vi "Lexer.vi"(8 "error in (no error)":errorcluster, 11 "Input":string) -> (0 "error out":errorcluster, 3 "Tokens":T1[](array[typedef]))   [LabVIEW 2022 SP3, in "Expressions.lvlib"]
uses:
  Expressions.lvlib
  Controls/Token.ctl
  Controls/Token Type.ctl
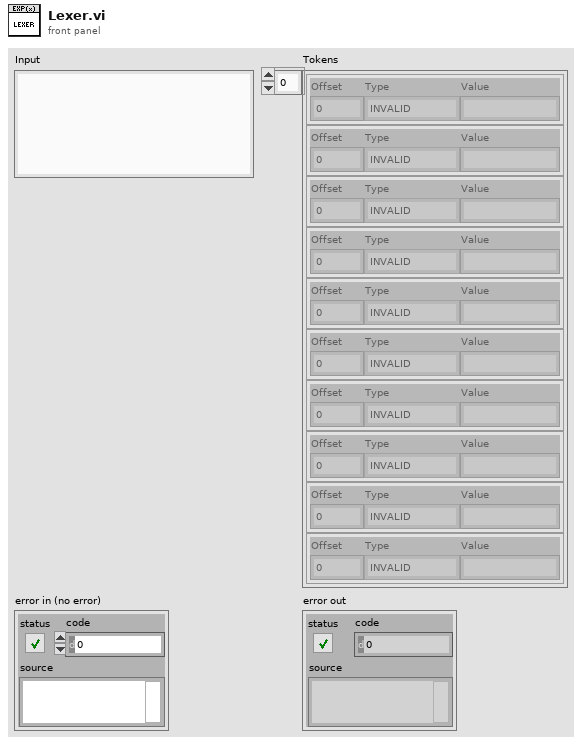
[diagram p1: front panel]
types:
  T1 = typedef "Expressions.lvlib/Token.ctl" = cluster{"Offset":i32, "Type":T2, "Value":string}
  T2 = typedef "Expressions.lvlib/Token Type.ctl" = enum8{"INVALID", "NOT", "AND", "OR", "EE", "NE", "LT", "GT", "LTE", "GTE", "PLUS", "MINUS", "MULTIPLY", "DIVIDE", "MODULUS", "LPAREN", "RPAREN", "LITERAL", "IDENTIFIER", "DEFINITION"}
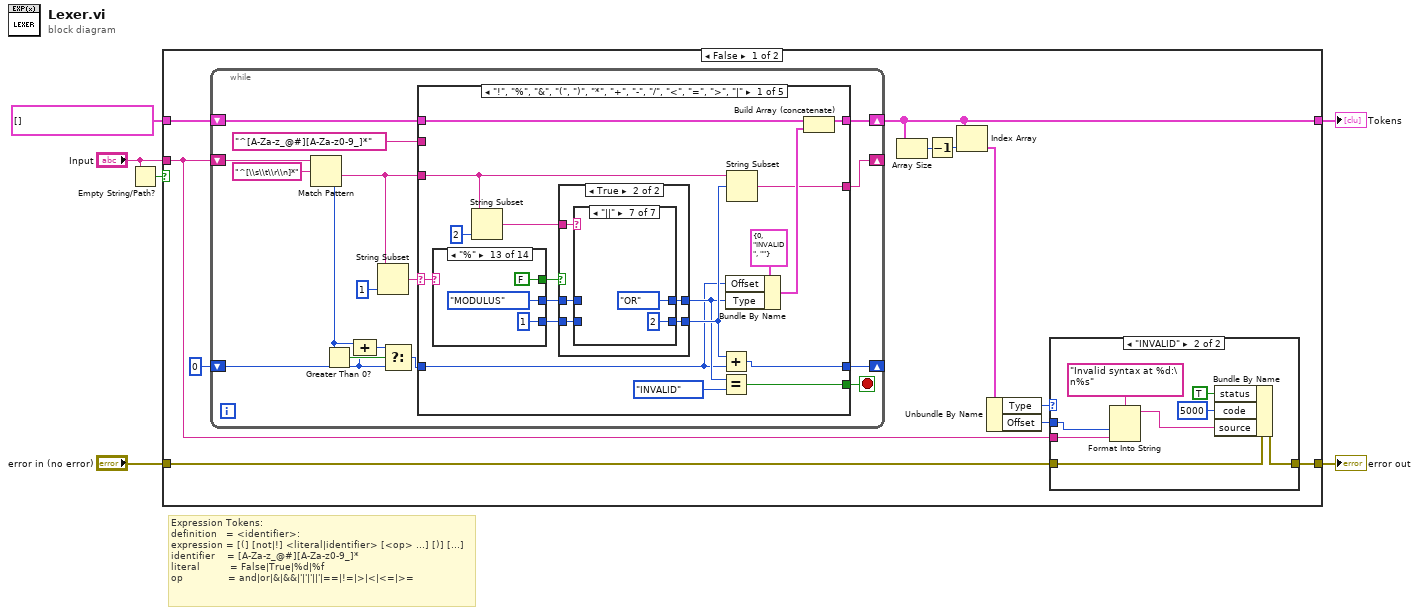
[diagram p0: block diagram]
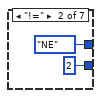
[diagram p5: hidden frame]
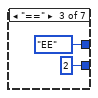
[diagram p6: hidden frame]
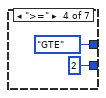
[diagram p7: hidden frame]
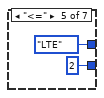
[diagram p8: hidden frame]
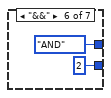
[diagram p9: hidden frame]
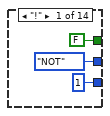
[diagram p10: hidden frame]
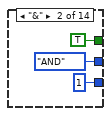
[diagram p11: hidden frame]
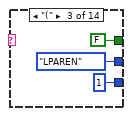
[diagram p12: hidden frame]
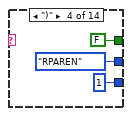
[diagram p13: hidden frame]
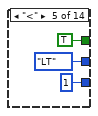
[diagram p14: hidden frame]
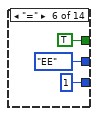
[diagram p15: hidden frame]
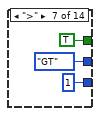
[diagram p16: hidden frame]
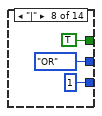
[diagram p17: hidden frame]
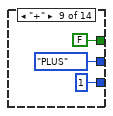
[diagram p18: hidden frame]
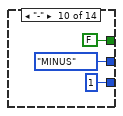
[diagram p19: hidden frame]
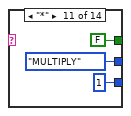
[diagram p20: hidden frame]
diagram:
  # "Expression Tokens:\ndefinition   = <identifier>:\nexpression = [(] [not|!] <literal|identifier> [<op> ...] [)] [...]\nidentifier    = [A-Za-z_@#][A-Za-z0-9_]*\nliteral          = False|True|%d|%f\nop               = and|or|&|&&|'|'|'||'|==|!=|>|<|<=|>="
  n1 = Empty String/Path?(string/path="Input") -> (empty?=w1:bool)
  n2 = case shown="False" w1 {
    tunnel: T1[] [] ("Tokens") -> [w17 w199]
    tunnel: "error in (no error)" -> [w15 w200]
    tunnel: [w14 w199] -> w4
    tunnel: [w11 w200] -> w3
    tunnel: "Input" -> [w8 _]
    frame False {
      n3 = while {
        shift-right: [w32] -> _
        shift-left: w8 -> [w42]
        shift-right: [w36] -> w14
        shift-left: w17 -> [w35]
        shift-right: [w28] -> _
        shift-left: 0 -> [w39]
        stop <- w33 stop-if-true
        n4 = Match Pattern(string=w42, regular expression="^[\\s\\t\\r\\n]*") -> (after substring=w31:string, offset past match=w38:i32)  [unwired: 1 in, 2 out]
        n5 = Greater Than 0?(x=w38) -> (x > 0?=w40:bool)
        n6 = Compound Arithmetic op=ADD(w38, w39) -> (w37:i32)
        n7 = String Subset(string=w31, length (rest)=1 ("length (rest)")) -> (substring=w29:string)  [unwired: 1 in]
        n8 = Select(t=w37, s=w40, f=w39) -> (s? t:f=w34:i32)
        n9 = case shown="\"!\", \"%\", \"&\", \"(\", \")\", \"*\", \"+\", \"-\", \"/\", \"<\", \"=\", \">\", \"|\"" w29 {
          selector: w29 -> [w47 _ _ _ _]
          tunnel: [w59 w137 w157 w189 w198] -> w36
          tunnel: w35 -> [w60 w138 w160 w190 w198]
          tunnel: w31 -> [w53 w129 w154 w180 _]
          tunnel: w34 -> [w43 w124 w149 w175 w196]
          tunnel: [w48 w132 _ w184 TRUE] -> w33
          tunnel: [w51 w127 w153 w177 _] -> w32
          tunnel: [w56 w134 w151 w186 w196] -> w28
          tunnel: "^[A-Za-z_@#][A-Za-z0-9_]*" ("regular expression") -> [_ w130 _ _ _]
          frame "!", "%", "&", "(", ")", "*", "+", "-", "/", "<", "=", ">", "|" {
            n10 = case shown="\"%\"" w47 {
              tunnel: [Token_Type."NOT" ("Token Type") Token_Type."AND" ("Token Type") Token_Type."LPAREN" ("Token Type") Token_Type."RPAREN" ("Token Type") Token_Type."LT" ("Token Type") Token_Type."EE" ("Token Type") Token_Type."GT" ("Token Type") Token_Type."OR" ("Token Type") Token_Type."PLUS" ("Token Type") Token_Type."MINUS" ("Token Type") Token_Type."MULTIPLY" ("Token Type") Token_Type."DIVIDE" ("Token Type") Token_Type."MODULUS" ("Token Type") Token_Type."INVALID" ("Token Type")] -> w44
              tunnel: [1 ("offset (0)") 1 ("offset (0)") 1 ("offset (0)") 1 ("offset (0)") 1 ("offset (0)") 1 ("offset (0)") 1 ("offset (0)") 1 ("offset (0)") 1 ("offset (0)") 1 ("offset (0)") 1 ("offset (0)") 1 ("offset (0)") 1 ("offset (0)") 0 ("offset (0)")] -> w45
              tunnel: [FALSE TRUE FALSE FALSE TRUE TRUE TRUE TRUE FALSE FALSE FALSE FALSE FALSE FALSE] -> w46
              frame "!" {
              }
              frame "&" {
              }
              frame "(" {
              }
              frame ")" {
              }
              frame "<" {
              }
              frame "=" {
              }
              frame ">" {
              }
              frame "|" {
              }
              frame "+" {
              }
              frame "-" {
              }
              frame "*" {
              }
              frame "/" {
              }
              frame "%" {
              }
              frame Default {
              }
            }
            n11 = String Subset(string=w53, length (rest)=2 ("offset (0)")) -> (substring=w54:string)  [unwired: 1 in]
            n12 = case shown="True" w46 {
              tunnel: w54 -> [_ w67]
              tunnel: [w62 w66] -> w52
              tunnel: [w61 w65] -> w50
              tunnel: w45 -> [w62 w64]
              tunnel: w44 -> [w61 w63]
              frame False {
              }
              frame True {
                n13 = case shown="\"||\"" w67 {
                  tunnel: [w68 Token_Type."NE" ("Token Type") Token_Type."EE" ("Token Type") Token_Type."GTE" ("Token Type") Token_Type."LTE" ("Token Type") Token_Type."AND" ("Token Type") Token_Type."OR" ("Token Type")] -> w65
                  tunnel: [w69 2 ("offset (0)") 2 ("offset (0)") 2 ("offset (0)") 2 ("offset (0)") 2 ("offset (0)") 2 ("offset (0)")] -> w66
                  tunnel: w64 -> [w69 _ _ _ _ _ _]
                  tunnel: w63 -> [w68 _ _ _ _ _ _]
                  frame Default {
                  }
                  frame "!=" {
                  }
                  frame "==" {
                  }
                  frame ">=" {
                  }
                  frame "<=" {
                  }
                  frame "&&" {
                  }
                  frame "||" {
                  }
                }
              }
            }
            n14 = Add(x=w52, y=w43) -> (x+y=w56:i32)
            n15 = Equal?(x=w50, y=Token_Type."INVALID") -> (x = y?=w48:bool)
            n16 = Bundle By Name(cluster=T1 {"Offset"=0, "Type"=enum."INVALID", "Value"=""} ("Token"), "Offset"=w43, "Type"=w50) -> (w57:T1)
            n17 = String Subset(string=w53, offset (0)=w52) -> (substring=w51:string)  [unwired: 1 in]
            n18 = Build Array (concatenate)(w60, w57) -> (w59:T1[])
          }
          frame "#", "@", "A".."Z", "_", "a".."z" {
            n19 = Match Pattern(string=w129, regular expression=w130) -> (match substring=w126:string, after substring=w127:string)  [unwired: 1 in, 2 out]
            n20 = case shown="\"False\", \"Inf\", \"NaN\", \"True\", \"and\", \"false\", \"inf\", \"nan\", \"not\", \"or\", \"true\"" w126 {
              selector: w126 -> [w140 w147]
              tunnel: [w141 Token_Type."IDENTIFIER" ("Token Type")] -> w131
              tunnel: [w139 w147] -> w128
              frame "False", "Inf", "NaN", "True", "and", "false", "inf", "nan", "not", "or", "true" {
                n21 = case shown="Default" w140 {
                  selector: w140 -> [_ _ _ w145]
                  tunnel: [Token_Type."AND" ("Token Type") Token_Type."OR" ("Token Type") Token_Type."NOT" ("Token Type") Token_Type."LITERAL" ("Token Type")] -> w141
                  tunnel: [_ _ _ w145] -> w139
                  frame "and" {
                  }
                  frame "or" {
                  }
                  frame "not" {
                  }
                  frame Default {
                  }
                }
              }
              frame Default {
              }
            }
            n22 = String Length(string=w126) -> (length=w125:i32)
            n23 = Add(x=w125, y=w124) -> (x+y=w134:i32)
            n24 = Equal?(x=w131, y=Token_Type."INVALID") -> (x = y?=w132:bool)
            n25 = Bundle By Name(cluster=T1 {"Offset"=0, "Type"=enum."INVALID", "Value"=""} ("Token"), "Offset"=w124, "Type"=w131, "Value"=w128) -> (w135:T1)
            n26 = Build Array (concatenate)(w138, w135) -> (w137:T1[])
          }
          frame ":" {
            # "<IDENTIFIER>: -> DEFINITION"
            n27 = Array Size(array=w160) -> (size(s)=w161:i32)
            n28 = Decrement(x=w161) -> (x-1=w158:i32)
            n29 = Index Array(array=w160, index=w158) -> (element=w159:T1)
            n30 = Unbundle By Name(w159) -> ("Type"=w156:T2)
            n31 = case shown="\"IDENTIFIER\"" w156 {
              tunnel: w160 -> [w167 w174]
              tunnel: w159 -> [_ w173]
              tunnel: w158 -> [_ w171]
              tunnel: [w166 w170] -> w157
              tunnel: Token_Type."DEFINITION" ("Type") -> [_ w169]
              tunnel: [0 1] -> w152
              tunnel: T1 {"Offset"=0, "Type"=enum."INVALID", "Value"=""} ("Token") -> [w165 _]
              tunnel: w149 -> [w163 _]
              frame Default {
                n32 = Bundle By Name(cluster=w165, "Offset"=w163) -> (w164:T1)
                n33 = Build Array (concatenate)(w167, w164) -> (w166:T1[])
              }
              frame "IDENTIFIER" {
                n34 = Bundle By Name(cluster=w173, "Type"=w169) -> (w172:T1)
                n35 = Replace Array Subset(array=w174, new element=w172, index=w171) -> (w170:T1[])
              }
            }
            n36 = Add(x=w152, y=w149) -> (x+y=w151:i32)
            n37 = String Subset(string=w154, offset (0)=w152) -> (substring=w153:string)  [unwired: 1 in]
          }
          frame Default {
            w181 = 0.0  # DBL
            # "%d, %f, -Inf"
            n38 = Fract/Exp String To Number(string=w180, default (0 dbl)=w181) -> (offset past number=w178:i32)  [unwired: 2 in, 1 out]
            n39 = String Subset(string=w180, length (rest)=w178) -> (substring=w179:string)  [unwired: 1 in]
            n40 = case shown="..0" w178 {
              selector: w178 -> [_ w194]
              tunnel: [Token_Type."INVALID" ("Token Type") Token_Type."LITERAL" ("Token Type")] -> w183
              tunnel: [_ w193] -> w182
              tunnel: [0 ("offset past number") w194] -> w176
              tunnel: w179 -> [_ w193]
              frame ..0 {
              }
              frame 1.. {
              }
            }
            n41 = String Subset(string=w180, offset (0)=w176) -> (substring=w177:string)  [unwired: 1 in]
            n42 = Bundle By Name(cluster=T1 {"Offset"=0, "Type"=enum."INVALID", "Value"=""} ("Token"), "Offset"=w175, "Type"=w183, "Value"=w182) -> (w187:T1)
            n43 = Add(x=w176, y=w175) -> (x+y=w186:i32)
            n44 = Equal?(x=w183, y=Token_Type."INVALID") -> (x = y?=w184:bool)
            n45 = Build Array (concatenate)(w190, w187) -> (w189:T1[])
          }
          frame "" {
          }
        }
      }
      n46 = Array Size(array=w14) -> (size(s)=w13:i32)
      n47 = Decrement(x=w13) -> (x-1=w10:i32)
      n48 = Index Array(array=w14, index=w10) -> (element=w12:T1)
      n49 = Unbundle By Name(w12) -> ("Type"=w9:T2, "Offset"=w7:i32)
      n50 = case shown="\"INVALID\"" w9 {
        tunnel: w15 -> [w18 w26]
        tunnel: [w18 w25] -> w11
        tunnel: w8 -> [_ w19]
        tunnel: w7 -> [_ w20]
        frame Default {
        }
        frame "INVALID" {
          n51 = Format Into String(format string="Invalid syntax at %d:\n%s" ("source"), w20, w19) -> (resulting string=w21:string)  [unwired: 2 in, 1 out]
          n52 = Bundle By Name(cluster=w26, "status"=TRUE, "code"=5000, "source"=w21) -> (w25:errorcluster)
        }
      }
    }
    frame True {
    }
  }
  "error out" <- w3
  "Tokens" <- w4
